vi "GetSiblings.vi"(8 "error in":errorcluster, 11 "node in":refnum<data-value>) -> (0 "error out":errorcluster, 3 "siblings":refnum<data-value>[](array[refnum]))   [LabVIEW 2025, in "CEF.lvlib" / "CEF_Node.lvclass"]
doc: "Copyright 2017 National Instruments Corporation\n\nLicensed under the Apache License, Version 2.0 (the \"License\"); you may not use this file except in compliance with the License. You may obtain a copy of the License at http://www.apache.org/licenses/LICENSE-2.0\nUnless required by applicable law or agreed to in writing, software distributed under the License is distributed on an \"AS IS\" BASIS, WITHOUT WARRANTIES OR CONDITIONS OF ANY KIND, either express or implied. See the License for the specific language governing permissions and limitations under the License."
uses:
  CEF_Node.lvclass
  CEF_Node.lvclass/CEF_Node.ctl
  ReadParent.vi
  ReadChildren.vi
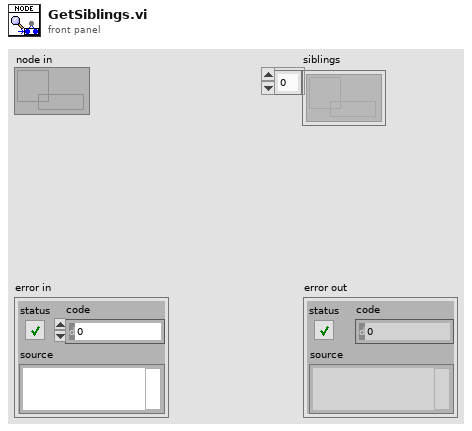
[diagram p1: front panel]
types:
  T1 = typedef "CEF.lvlib/CEF_Node.lvclass/NodeRef.ctl" = refnum<data-value>
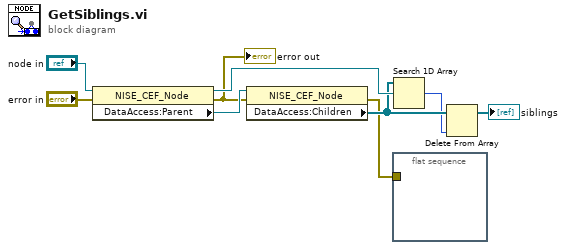
[diagram p0: block diagram]
diagram:
  n1 = property class="NISE_CEF_Node"(reference="node in", error in="error in") -> (reference out=w6:refnum<data-value>, error out=w1:errorcluster, "DataAccess:Parent"=w7:T1)
  "error out" <- w1
  n2 = property class="NISE_CEF_Node"(reference=w7, error in=w1) -> (error out=w2:errorcluster, "DataAccess:Children"=w5:T1[])  [unwired: 1 out]
  n3 = flat-sequence {
    tunnel: w2 -> [_]
    frame #0 {
    }
  }
  n4 = Search 1D Array(1D array=w5, element=w6) -> (index of element=w3:i32)  [unwired: 1 in]
  n5 = Delete From Array(array=w5, index=w3) -> (array with subset deleted=→"siblings":T1[])  [unwired: 1 in, 1 out]
